vi "final.vi"   [LabVIEW 2018]
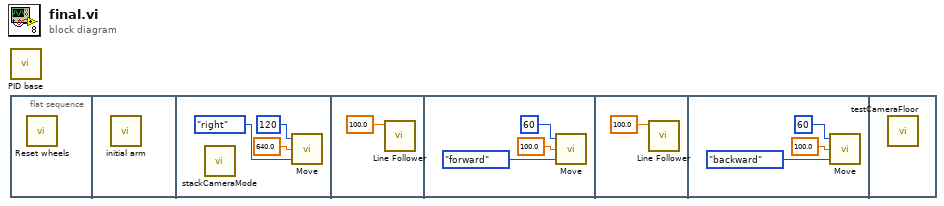
[diagram p0: block diagram]
diagram:
  n1 = call "PID base.vi"() -> ()  [unwired: 12 in]
  n2 = flat-sequence {
    frame #0 {
      n3 = call "Reset wheels.vi"() -> ()  [unwired: 12 in]
    }
    frame #1 {
      n4 = call "initial arm.vi"() -> ()  [unwired: 12 in]
    }
    frame #2 {
      n5 = call "stackCameraMode.vi"() -> ()  [unwired: 12 in]
      n6 = call "Move.vi"("Enum"=enum16{"forward", "backward", "left", "right"}."right", "distance"=640.0, "speed"=120) -> ()  [unwired: 1 in]
    }
    frame #3 {
      n7 = call "Line Follower.vi"("speed"=100.0) -> ()  [unwired: 11 in]
    }
    frame #4 {
      n8 = call "Move.vi"("Enum"=enum16{"forward", "backward", "left", "right"}."forward", "distance"=100.0, "speed"=60) -> ()  [unwired: 1 in]
    }
    frame #5 {
      n9 = call "Line Follower.vi"("speed"=100.0) -> ()  [unwired: 11 in]
    }
    frame #6 {
      n10 = call "Move.vi"("Enum"=enum16{"forward", "backward", "left", "right"}."backward", "distance"=100.0, "speed"=60) -> ()  [unwired: 1 in]
    }
    frame #7 {
      n11 = call "testCameraFloor.vi"() -> ()  [unwired: 12 in]
    }
  }
